vi "PAM uPa per Bit.vi"() -> ()   [LabVIEW 2020, in "PAM Library.lvlib"]
uses:
  PAM Library.lvlib
panel:
  out "uPa per Bit":dbl
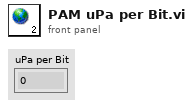
[diagram p1: front panel]
diagram:
